vi "Write new_plays.vi"(8 "error in (no error)":errorcluster, 10 "new_plays":T1, 11 "Playbook in":refnum<class "Playbook.lvclass">) -> (0 "error out":errorcluster, 3 "Playbook out":refnum<class "Playbook.lvclass">)   [LabVIEW 2022 SP3, in "Playbook.lvclass"]
uses:
  Playbook.lvclass
  NewOff1/NewOff1.lvclass
  Playbook.lvclass/Playbook.ctl
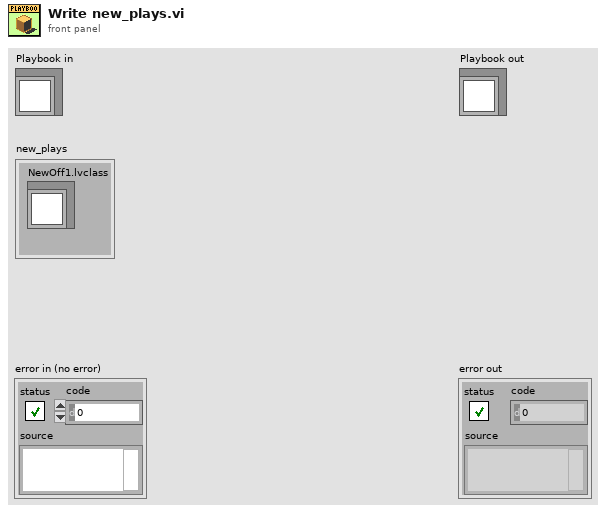
[diagram p1: front panel]
types:
  T1 = cluster{"NewOff1.lvclass":refnum<class "NewOff1.lvclass">}
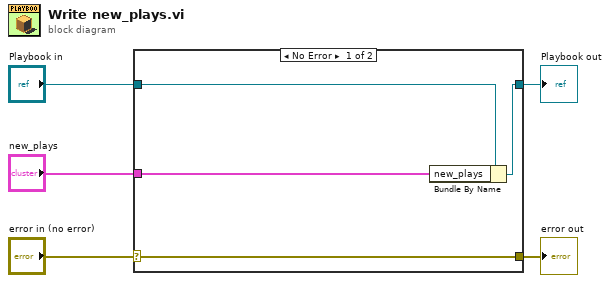
[diagram p0: block diagram]
diagram:
  n1 = case shown="No Error" "error in (no error)" {
    selector: "error in (no error)" -> [w9 w10]
    tunnel: [w9 w10] -> w4
    tunnel: [w7 w11] -> w2
    tunnel: "Playbook in" -> [w8 w11]
    tunnel: "new_plays" -> [w6 _]
    frame No Error {
      n2 = Bundle By Name(cluster=w8, "new_plays"=w6) -> (w7:refnum<class "Playbook.lvclass">)
    }
    frame Error {
    }
  }
  "error out" <- w4
  "Playbook out" <- w2
